vi "Resave_Non-affected_Subtrack_(11)-1.vi"(6 "[IN] Index for Not\nAffected Track":i32, 8 "error IN":errorcluster, 9 "[IN] Index of recon\nstructed tracks":i32, 10 "[IN] Clusters for Re\nconstructed Tracks":T1, 11 "[IN] Still connected\ntracks in group":T2) -> (0 "error OUT":errorcluster, 2 "[OUT] Clusters for Re\nconstructed Tracks":T1)   [LabVIEW 2013]
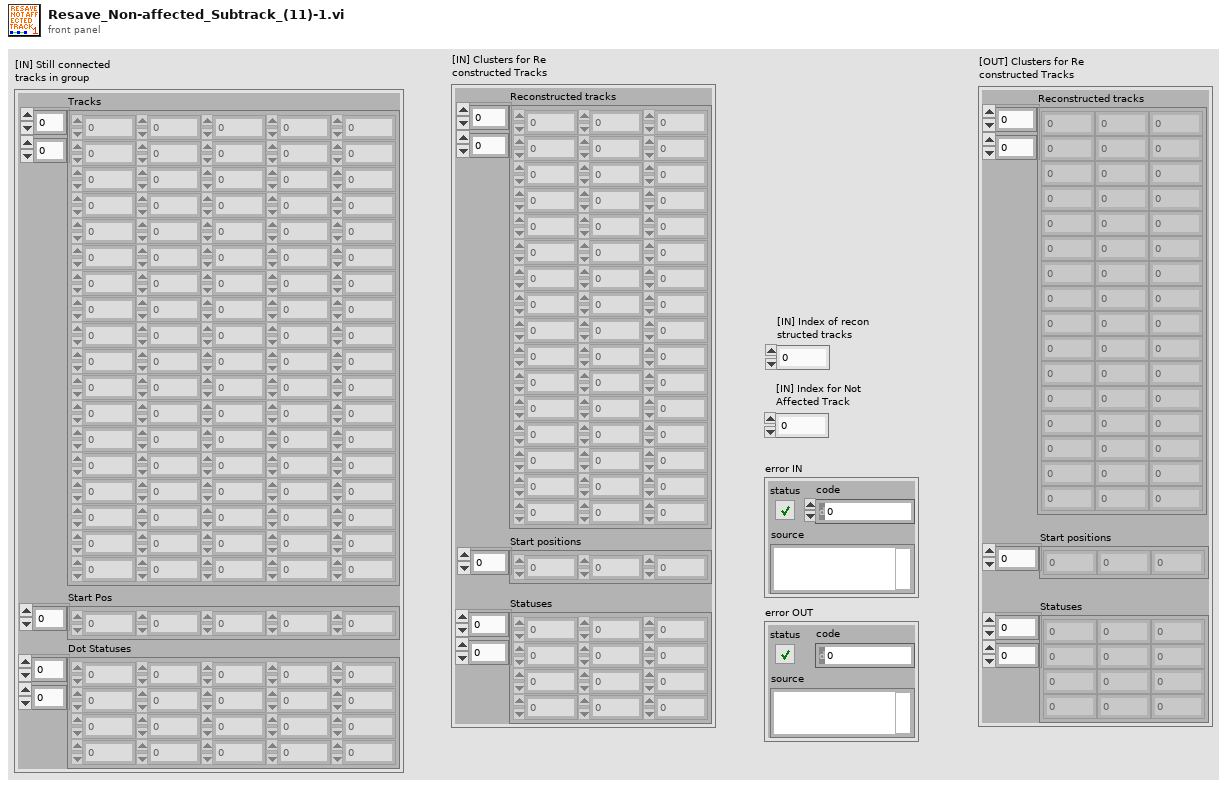
[diagram p1: front panel]
types:
  T1 = cluster{"Reconstructed tracks":dbl[][], "Start positions":i32[], "Statuses":i16[][]}
  T2 = cluster{"Tracks":dbl[][], "Start Pos":i32[], "Dot Statuses":i16[][]}
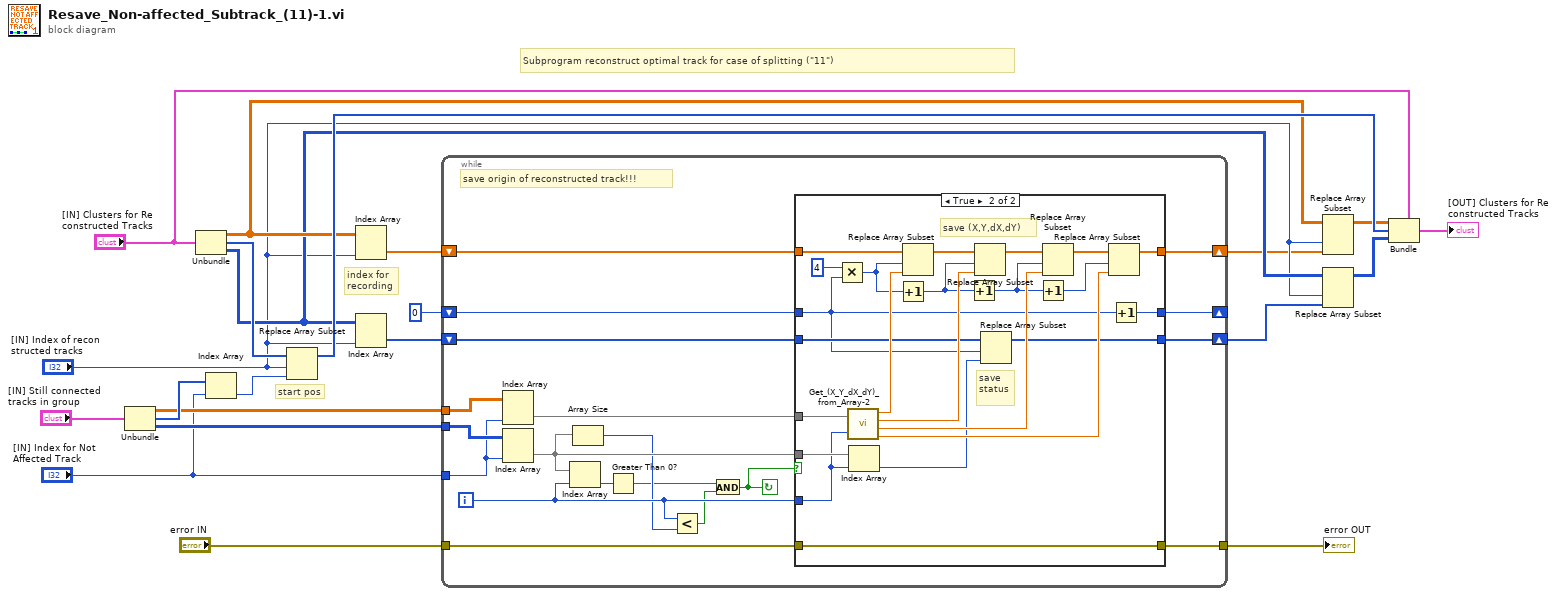
[diagram p0: block diagram]
diagram:
  # "Subprogram reconstruct optimal track for case of splitting (\"11\")"
  # "index for\nrecording"
  # "start pos"
  n1 = Unbundle("[IN] Still connected\ntracks in group") -> ("Tracks"=w15:dbl[][], "Start Pos"=w20:i32[], "Dot Statuses"=w5:i16[][])
  n2 = Unbundle("[IN] Clusters for Re\nconstructed Tracks") -> ("Reconstructed tracks"=w12:dbl[][], "Start positions"=w21:i32[], "Statuses"=w10:i16[][])
  n3 = Index Array(array=w20, index="[IN] Index for Not\nAffected Track") -> (element=w19:i32)
  n4 = Replace Array Subset(array=w21, new element=w19, index="[IN] Index of recon\nstructed tracks") -> (w13:i32[])
  n5 = Index Array(array=w12, index (col)="[IN] Index of recon\nstructed tracks") -> (element=w18:dbl[])  [unwired: 1 in]
  n6 = Index Array(array=w10, index (col)="[IN] Index of recon\nstructed tracks") -> (element=w17:i16[])  [unwired: 1 in]
  n7 = while {
    tunnel: w15 -> [w41]
    tunnel: w5 -> [w40]
    tunnel: "[IN] Index for Not\nAffected Track" -> [w39]
    shift-right: [w34] -> w3
    shift-left: w18 -> [w38]
    shift-right: [w32] -> w2
    shift-left: w17 -> [w36]
    shift-right: [w33] -> _
    shift-left: 0 -> [w35]
    tunnel: "error IN" -> [w31]
    tunnel: [w30] -> w1
    i -> [w27]
    stop <- w23 continue-if-true
    # "save origin of reconstructed track!!!"
    n8 = Index Array(array=w41, index (col)=w39) -> (element=w37:dbl[])  [unwired: 1 in]
    n9 = Index Array(array=w40, index (col)=w39) -> (element=w28:i16[])  [unwired: 1 in]
    n10 = Index Array(array=w28, index=w27) -> (element=w29:i16)
    n11 = Array Size(array=w28) -> (size(s)=w26:i32)
    n12 = Greater Than 0?(x=w29) -> (x > 0?=w25:bool)
    n13 = Less?(x=w27, y=w26) -> (x < y?=w24:bool)
    n14 = And(x=w25, y=w24) -> (x .and. y?=w23:bool)
    n15 = case shown="True" w23 {
      tunnel: w38 -> [w45 w66]
      tunnel: w37 -> [_ w68]
      tunnel: w28 -> [_ w67]
      tunnel: w27 -> [_ w51]
      tunnel: w36 -> [w43 w53]
      tunnel: [w43 w50] -> w32
      tunnel: [w45 w49] -> w34
      tunnel: w35 -> [w44 w48]
      tunnel: [w44 w47] -> w33
      tunnel: w31 -> [w42 w46]
      tunnel: [w42 w46] -> w30
      frame False {
      }
      frame True {
        # "save (X,Y,dX,dY)"
        # "save\nstatus"
        n16 = Multiply(x=4, y=w48) -> (x*y=w62:i32)
        n17 = call "Get_(X_Y_dX_dY)_from_Array-2.vi"("(X,Y,dX,dY)"=w68, "Index of Displacement"=w51) -> ("X"=w64:dbl, "Y"=w61:dbl, "dX"=w58:dbl, "dY"=w54:dbl)
        n18 = Index Array(array=w67, index=w51) -> (element=w52:i16)
        n19 = Increment(x=w62) -> (x+1=w59:i32)
        n20 = Replace Array Subset(array=w66, new element=w64, index=w62) -> (w63:dbl[])
        n21 = Increment(x=w59) -> (x+1=w57:i32)
        n22 = Replace Array Subset(array=w63, new element=w61, index=w59) -> (w60:dbl[])
        n23 = Replace Array Subset(array=w53, new element=w52, index=w48) -> (w50:i16[])
        n24 = Increment(x=w57) -> (x+1=w56:i32)
        n25 = Replace Array Subset(array=w60, new element=w58, index=w57) -> (w55:dbl[])
        n26 = Replace Array Subset(array=w55, new element=w54, index=w56) -> (w49:dbl[])
        n27 = Increment(x=w48) -> (x+1=w47:i32)
      }
    }
  }
  "error OUT" <- w1
  n28 = Replace Array Subset(array=w12, new element=w3, index (col)="[IN] Index of recon\nstructed tracks") -> (w11:dbl[][])  [unwired: 1 in]
  n29 = Replace Array Subset(array=w10, new element=w2, index (col)="[IN] Index of recon\nstructed tracks") -> (w8:i16[][])  [unwired: 1 in]
  n30 = Bundle(cluster="[IN] Clusters for Re\nconstructed Tracks", "Reconstructed tracks"=w11, "Start positions"=w13, "Statuses"=w8) -> (→"[OUT] Clusters for Re\nconstructed Tracks":T1)
